vi "CPU_only.vi"() -> ()   [LabVIEW 2019]
uses:
  <vilib>/Analysis/baseanly.llb/Real Inverse Matrix.vi
  <vilib>/Analysis/Matrix/Numeric/Multiply/Multiply - RM,RM.vi
  <vilib>/Analysis/Matrix/Numeric/Add/Add - RM,RM.vi
  <vilib>/Analysis/7linalg.llb/Real Eigenvalues and Vectors.vi
  <vilib>/Analysis/NI_AALBase.lvlib
  <vilib>/Analysis/Matrix/NI_Matrix.lvlib
  <vilib>/Analysis/NI_AALPro.lvlib
panel:
  out "Frequencies":dbl[](array[numeric])
  out "Run Time (ms)":u32 format="%_6f"
  out "Eigenvalues":cdb[][](array[numeric]) format="%#_4g"
  out "K input":dbl[][](array[numeric])
  out "M input":dbl[][](array[numeric])
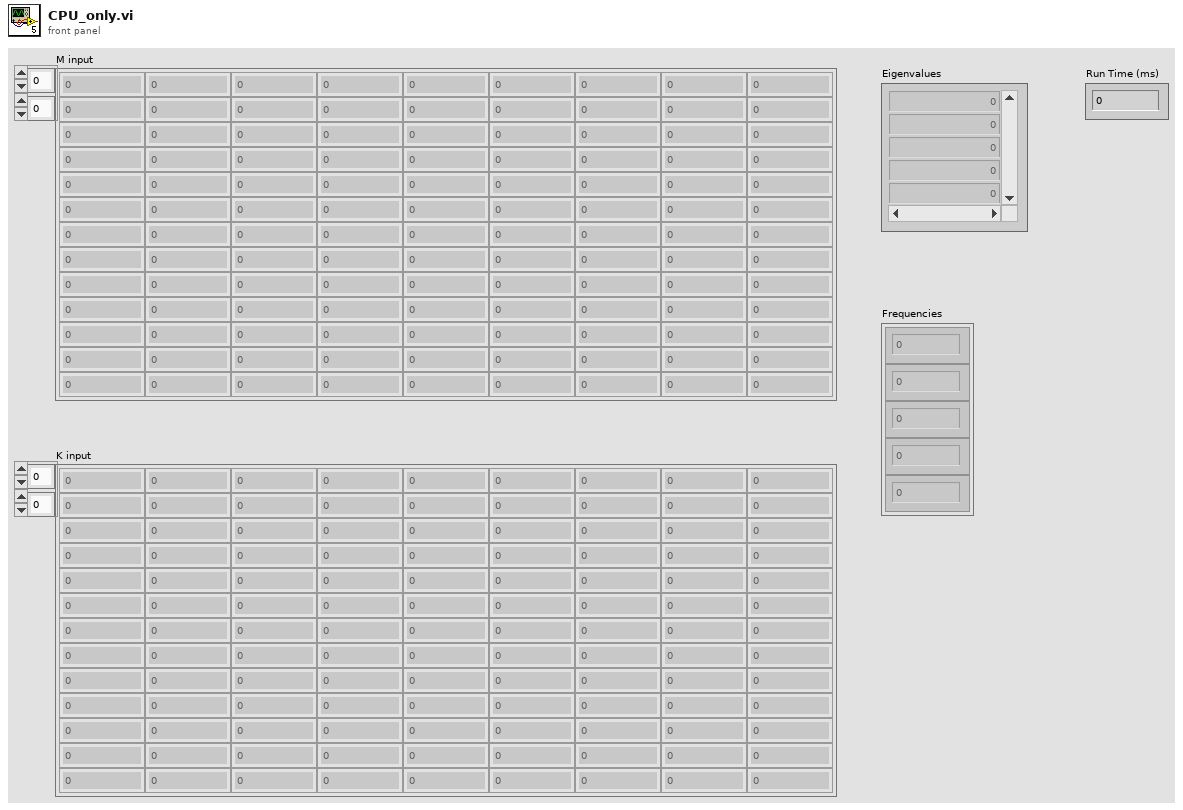
[diagram p1: front panel]
types:
  T1 = typedef "NI_Matrix.lvlib/RealMatrix.ctl" = dbl[][]
  T2 = typedef "NI_Matrix.lvlib/ComplexMatrix.ctl" = cdb[][]
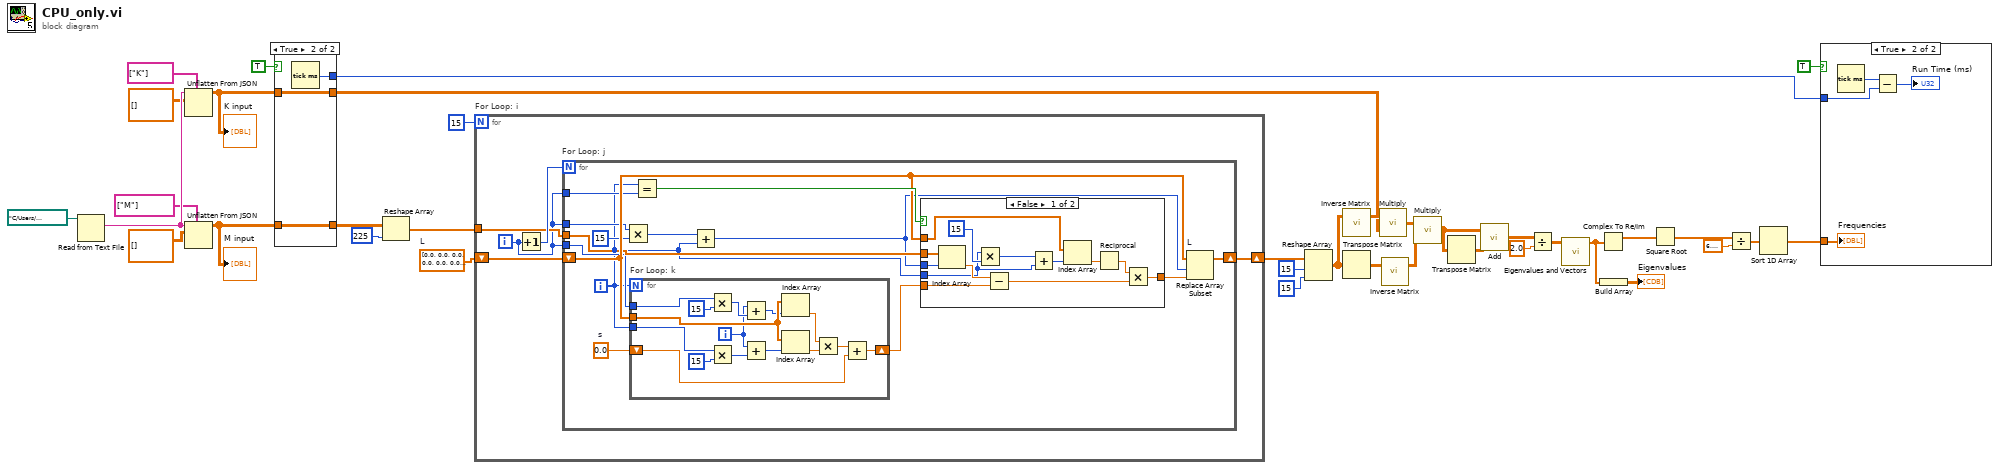
[diagram p0: block diagram]
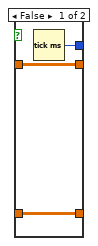
[diagram p3: hidden frame]
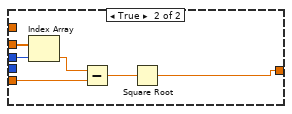
[diagram p4: hidden frame]
diagram:
  w37 = sgl[] [0.0, 0.0, 0.0, 0.0, 0.0, 0.0, 0.0, 0.0, 0.0, 0.0, 0.0, 0.0, 0.0, 0.0, 0.0, 0.0, 0.0, 0.0, 0.0, 0.0, 0.0, 0.0, 0.0, 0.0, 0.0, 0.0, 0.0, 0.0, 0.0, 0.0, 0.0, 0.0, 0.0, 0.0, 0.0, 0.0, 0.0, 0.0, 0.0, 0.0, 0.0, 0.0, 0.0, 0.0, 0.0, 0.0, 0.0, 0.0, 0.0, 0.0, 0.0, 0.0, 0.0, 0.0, 0.0, 0.0, 0.0, 0.0, 0.0, 0.0, 0.0, 0.0, 0.0, 0.0, 0.0, 0.0, 0.0, 0.0, 0.0, 0.0, 0.0, 0.0, 0.0, 0.0, 0.0, 0.0, 0.0, 0.0, 0.0, 0.0, 0.0, 0.0, 0.0, 0.0, 0.0, 0.0, 0.0, 0.0, 0.0, 0.0, 0.0, 0.0, 0.0, 0.0, 0.0, 0.0, 0.0, 0.0, 0.0, 0.0, 0.0, 0.0, 0.0, 0.0, 0.0, 0.0, 0.0, 0.0, 0.0, 0.0, 0.0, 0.0, 0.0, 0.0, 0.0, 0.0, 0.0, 0.0, 0.0, 0.0, 0.0, 0.0, 0.0, 0.0, 0.0, 0.0, 0.0, 0.0, 0.0, 0.0, 0.0, 0.0, 0.0, 0.0, 0.0, 0.0, 0.0, 0.0, 0.0, 0.0, 0.0, 0.0, 0.0, 0.0, 0.0, 0.0, 0.0, 0.0, 0.0, 0.0, 0.0, 0.0, 0.0, 0.0, 0.0, 0.0, 0.0, 0.0, 0.0, 0.0, 0.0, 0.0, 0.0, 0.0, 0.0, 0.0, 0.0, 0.0, 0.0, 0.0, 0.0, 0.0, 0.0, 0.0, 0.0, 0.0, 0.0, 0.0, 0.0, 0.0, 0.0, 0.0, 0.0, 0.0, 0.0, 0.0, 0.0, 0.0, 0.0, 0.0, 0.0, 0.0, 0.0, 0.0, 0.0, 0.0, 0.0, 0.0, 0.0, 0.0, 0.0, 0.0, 0.0, 0.0, 0.0, 0.0, 0.0, 0.0, 0.0, 0.0, 0.0, 0.0, 0.0, 0.0, 0.0, 0.0, 0.0, 0.0, 0.0, 0.0, 0.0, 0.0, 0.0, 0.0, 0.0]  # L
  n1 = Read from Text File(file (use dialog)=path "C:/Users/PXIe-8880/Documents/AFRL_summer_2019/Cholesky_FPGA/Cholesky_FPGA_V1/data/data.txt") -> (text=w33:string)  [unwired: 3 in, 3 out]
  n2 = Unflatten From JSON(path=string[] ["K"], JSON string=w33, type and defaults=dbl[][] []) -> (value=w35:dbl[][])  [unwired: 4 in, 1 out]
  "K input" <- w35
  n3 = Unflatten From JSON(path=string[] ["M"], JSON string=w33, type and defaults=dbl[][] []) -> (value=w34:dbl[][])  [unwired: 4 in, 1 out]
  "M input" <- w34
  n4 = case shown="True" TRUE {
    tunnel: w34 -> [w40 w43]
    tunnel: [w40 w43] -> w25
    tunnel: w35 -> [w39 w42]
    tunnel: [w39 w42] -> w3
    tunnel: [w38 w41] -> w1
    frame False {
      n5 = Tick Count (ms)() -> (millisecond timer value=w38:u32)
    }
    frame True {
      n6 = Tick Count (ms)() -> (millisecond timer value=w41:u32)
    }
  }
  n7 = Reshape Array(w25, 225 ("dimension size")) -> (w24:dbl[])
  n8 = for "For Loop: i" {
    N: 15 -> [_]
    shift-right: [w46] -> w5
    shift-left: w37 -> [w48]
    tunnel: w24 -> [w45]
    i -> [w44]
    n9 = Increment(x=w44) -> (x+1=w47:i32)
    n10 = for "For Loop: j" {
      N: w47 -> [_]
      tunnel: w44 -> [w56]
      shift-right: [w58] -> w46
      shift-left: w48 -> [w57]
      tunnel: w44 -> [w55]
      tunnel: w45 -> [w52]
      tunnel: w44 -> [w50]
      i -> [w49]
      w61 = sgl 0.0  # s
      n11 = Multiply(x=w55, y=15) -> (x*y=w53:i32)
      n12 = for "For Loop: k" {
        N: w49 -> [_]
        tunnel: w57 -> [w95]
        shift-right: [w91] -> w60
        shift-left: w61 -> [w92]
        tunnel: w50 -> [w90]
        tunnel: w49 -> [w83]
        i -> [w82]
        n13 = Multiply(x=w90, y=15) -> (x*y=w88:i32)
        n14 = Multiply(x=w83, y=15) -> (x*y=w85:i32)
        n15 = Add(x=w82, y=w88) -> (x+y=w87:i32)
        n16 = Add(x=w82, y=w85) -> (x+y=w84:i32)
        n17 = Index Array(array=w95, index=w87) -> (element=w96:sgl)
        n18 = Index Array(array=w95, index=w84) -> (element=w94:sgl)
        n19 = Multiply(x=w96, y=w94) -> (x*y=w93:sgl)
        n20 = Add(x=w93, y=w92) -> (x+y=w91:sgl)
      }
      n21 = Equal?(x=w49, y=w56) -> (x = y?=w62:bool)
      n22 = Add(x=w53, y=w49) -> (x+y=w51:i32)
      n23 = case shown="False" w62 {
        tunnel: w60 -> [w73 w81]
        tunnel: [w72 w79] -> w59
        tunnel: w57 -> [w75 _]
        tunnel: w52 -> [w69 w78]
        tunnel: w51 -> [w68 w77]
        tunnel: w49 -> [w64 _]
        frame False {
          n24 = Index Array(array=w69, index=w68) -> (element=w67:dbl)
          n25 = Multiply(x=w64, y=15) -> (x*y=w65:i32)
          n26 = Subtract(x=w67, y=w73) -> (x-y=w70:dbl)
          n27 = Add(x=w65, y=w64) -> (x+y=w63:i32)
          n28 = Index Array(array=w75, index=w63) -> (element=w74:sgl)
          n29 = Reciprocal(x=w74) -> (1/x=w71:sgl)
          n30 = Multiply(x=w71, y=w70) -> (x*y=w72:dbl)
        }
        frame True {
          n31 = Index Array(array=w78, index=w77) -> (element=w76:dbl)
          n32 = Subtract(x=w76, y=w81) -> (x-y=w80:dbl)
          n33 = Square Root(x=w80) -> (sqrt(x)=w79:dbl)
        }
      }
      n34 = Replace Array Subset "L"(array=w57, new element=w59, index=w51) -> (w58:sgl[])
    }
  }
  n35 = Reshape Array(w5, 15 ("dimension size"), 15 ("dimension size")) -> (w4:sgl[][])
  n36 = call-poly <vilib>:"Inverse Matrix.vi"("Input Matrix"=w4) -> ("Inverse Matrix"=w14:T1)  [unwired: 1 in, 1 out]
  n37 = Transpose Matrix(1:w4) -> (0:w6:dbl[][])
  n38 = call-poly <vilib>:"Multiply.vi"("Real Matrix B"=w3, "Real Matrix A"=w14) -> ("A * B"=w12:T1)
  n39 = call-poly <vilib>:"Inverse Matrix.vi"("Input Matrix"=w6) -> ("Inverse Matrix"=w13:T1)  [unwired: 1 in, 1 out]
  n40 = call-poly <vilib>:"Multiply.vi"("Real Matrix B"=w13, "Real Matrix A"=w12) -> ("A * B"=w11:T1)
  n41 = Transpose Matrix(1:w11) -> (0:w10:T1)
  n42 = call-poly <vilib>:"Add.vi"("Real Matrix B"=w10, "Real Matrix A"=w11) -> ("A + B"=w8:T1)
  n43 = Divide(x=w8, y=2.0) -> (x/y=w7:T1)
  n44 = call-poly <vilib>:"Eigenvalues and Vectors.vi"("Input Matrix"=w7) -> ("Eigenvalues"=w2:cdb[])  [unwired: 2 in, 2 out]
  n45 = Complex To Re/Im ("Complex To Cartesian.vi")(x + iy=w2) -> (x=w20:dbl[])  [unwired: 1 out]
  n46 = Build Array(w2) -> (→"Eigenvalues":T2)
  n47 = Square Root ("Square Root.vi")(x=w20) -> (sqrt(x)=w21:dbl[])
  n48 = Divide(x=w21, y=6.283185307179586) -> (x/y=w22:dbl[])
  n49 = Sort 1D Array(array=w22) -> (sorted array=w23:dbl[])
  n50 = case shown="True" TRUE {
    tunnel: w23 -> [_ w100]
    tunnel: w1 -> [_ w97]
    frame False {
    }
    frame True {
      n51 = Tick Count (ms)() -> (millisecond timer value=w99:u32)
      n52 = Subtract(x=w99, y=w97) -> (x-y=→"Run Time (ms)":u32)
      "Frequencies" <- w100
    }
  }
